vi "ContPreProc_old.vi"(8 "Step In":dbl, 10 "Compiler Settings":T1={"Python Path"=path "", "Main File"="makesequence.py", "Meta File"="makesequence.py", "Aux File"="C:\\Python27"}, 11 "Master Exp In":T2) -> (2 "Aux Pulse Out":T4, 3 "Main Pulse Out":T4)   [LabVIEW 2017]
uses:
  PulseControl.ctl
  Compiler/Params.ctl
  PulseCompiler/SequenceCluster.ctl
  controls/MasterExperiment.ctl
  PulseCompiler/CompilerSettings.ctl
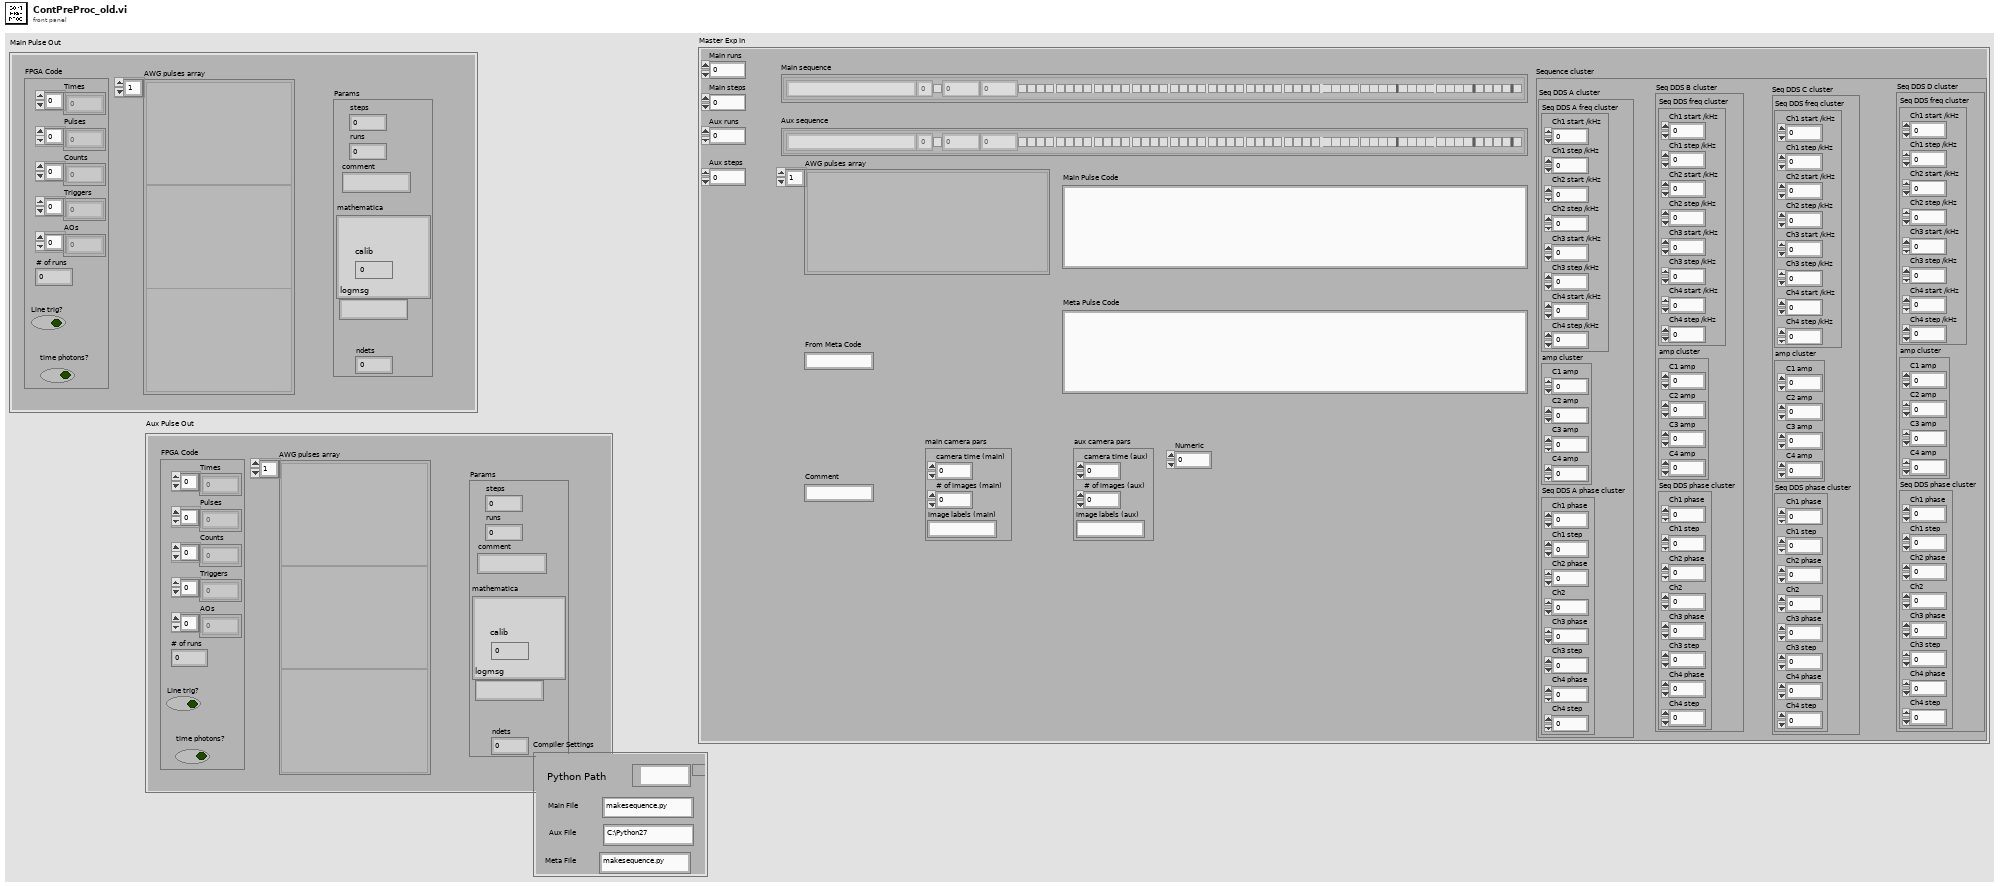
[diagram p1: front panel]
types:
  T1 = typedef "CompilerSettings.ctl" = cluster{"Python Path":path, "Main File":string, "Meta File":string, "Aux File":string}
  T2 = typedef "MasterExperiment.ctl" = cluster{"Main runs":dbl, "Numeric":dbl, "Main steps":dbl, "Aux runs":dbl, "Aux steps":dbl, "Main sequence":cluster{"Pulse name":string, "Pulse number":i32, "Enabled?":bool, "Time":dbl, "Step":dbl, "Pulse 0":bool, "Pulse 1":bool, "Pulse 2":bool, "Pulse 3":bool, "Pulse 4":bool, "Pulse 5":bool, "Pulse 6":bool, "Pulse 7":bool, "Pulse 8":bool, "Pulse 9":bool, "Pulse 10":bool, "Pulse 11":bool, "Pulse 12":bool, "Pulse 13":bool, "Pulse 14":bool, "Pulse 15":bool, "Pulse 16":bool, "Pulse 17":bool, "Pulse 18":bool, "Pulse 19":bool, "Pulse 20":bool, "Pulse 21":bool, "Pulse 22":bool, "Pulse 23":bool, "Pulse 24":bool, "Pulse 25":bool, "Pulse 26":bool, "Pulse 27":bool, "Pulse 28":bool, "Pulse 29":bool, "Pulse 30":bool, "Pulse 31":bool, "Pulse 32":bool, "Pulse 33":bool, "Pulse 34":bool, "Pulse 35":bool, "Pulse 36":bool, "Pulse 37":bool, "Pulse 38":bool, "Pulse 39":bool, "Count 0":bool, "Count 1":bool, "Count 2":bool, "Count 3":bool, "Count 4":bool, "Count 5":bool, "Count 6":bool, "Count 7":bool, "AO 0":bool, "AO 1":bool, "AO 2":bool, "AO 3":bool, "Trigger 0":bool}[], "Aux sequence":cluster{"Pulse name":string, "Pulse number":i32, "Enabled?":bool, "Time":dbl, "Step":dbl, "Pulse 0":bool, "Pulse 1":bool, "Pulse 2":bool, "Pulse 3":bool, "Pulse 4":bool, "Pulse 5":bool, "Pulse 6":bool, "Pulse 7":bool, "Pulse 8":bool, "Pulse 9":bool, "Pulse 10":bool, "Pulse 11":bool, "Pulse 12":bool, "Pulse 13":bool, "Pulse 14":bool, "Pulse 15":bool, "Pulse 16":bool, "Pulse 17":bool, "Pulse 18":bool, "Pulse 19":bool, "Pulse 20":bool, "Pulse 21":bool, "Pulse 22":bool, "Pulse 23":bool, "Pulse 24":bool, "Pulse 25":bool, "Pulse 26":bool, "Pulse 27":bool, "Pulse 28":bool, "Pulse 29":bool, "Pulse 30":bool, "Pulse 31":bool, "Pulse 32":bool, "Pulse 33":bool, "Pulse 34":bool, "Pulse 35":bool, "Pulse 36":bool, "Pulse 37":bool, "Pulse 38":bool, "Pulse 39":bool, "Count 0":bool, "Count 1":bool, "Count 2":bool, "Count 3":bool, "Count 4":bool, "Count 5":bool, "Count 6":bool, "Count 7":bool, "AO 0":bool, "AO 1":bool, "AO 2":bool, "AO 3":bool, "Trigger 0":bool}[], "AWG pulses array":variant[], "Main Pulse Code":string, "Meta Pulse Code":string, "Comment":string, "main camera pars":cluster{"camera time (main)":i32, "# of images (main)":i32, "image labels (main)":string}, "aux camera pars":cluster{"camera time (aux)":i32, "# of images (aux)":i32, "image labels (aux)":string}, "From Meta Code":string, "Sequence cluster":T3}
  T3 = typedef "SequenceCluster.ctl" = cluster{"Seq DDS A cluster":cluster{"Seq DDS A freq cluster":cluster{"Ch1 start /kHz":dbl, "Ch1 step /kHz":dbl, "Ch2 start /kHz":dbl, "Ch2 step /kHz":dbl, "Ch3 start /kHz":dbl, "Ch3 step /kHz":dbl, "Ch4 start /kHz":dbl, "Ch4 step /kHz":dbl}, "amp cluster":cluster{"C1 amp":dbl, "C2 amp":dbl, "C3 amp":dbl, "C4 amp":dbl}, "Seq DDS A phase cluster":cluster{"Ch1 phase":dbl, "Ch1 step":dbl, "Ch2 phase":dbl, "Ch2":dbl, "Ch3 phase":dbl, "Ch3 step":dbl, "Ch4 phase":dbl, "Ch4 step":dbl}}, "Seq DDS B cluster":cluster{"Seq DDS freq cluster":cluster{"Ch1 start /kHz":dbl, "Ch1 step /kHz":dbl, "Ch2 start /kHz":dbl, "Ch2 step /kHz":dbl, "Ch3 start /kHz":dbl, "Ch3 step /kHz":dbl, "Ch4 start /kHz":dbl, "Ch4 step /kHz":dbl}, "amp cluster":cluster{"C1 amp":dbl, "C2 amp":dbl, "C3 amp":dbl, "C4 amp":dbl}, "Seq DDS phase cluster":cluster{"Ch1 phase":dbl, "Ch1 step":dbl, "Ch2 phase":dbl, "Ch2":dbl, "Ch3 phase":dbl, "Ch3 step":dbl, "Ch4 phase":dbl, "Ch4 step":dbl}}, "Seq DDS C cluster":cluster{"Seq DDS freq cluster":cluster{"Ch1 start /kHz":dbl, "Ch1 step /kHz":dbl, "Ch2 start /kHz":dbl, "Ch2 step /kHz":dbl, "Ch3 start /kHz":dbl, "Ch3 step /kHz":dbl, "Ch4 start /kHz":dbl, "Ch4 step /kHz":dbl}, "amp cluster":cluster{"C1 amp":dbl, "C2 amp":dbl, "C3 amp":dbl, "C4 amp":dbl}, "Seq DDS phase cluster":cluster{"Ch1 phase":dbl, "Ch1 step":dbl, "Ch2 phase":dbl, "Ch2":dbl, "Ch3 phase":dbl, "Ch3 step":dbl, "Ch4 phase":dbl, "Ch4 step":dbl}}, "Seq DDS D cluster":cluster{"Seq DDS freq cluster":cluster{"Ch1 start /kHz":dbl, "Ch1 step /kHz":dbl, "Ch2 start /kHz":dbl, "Ch2 step /kHz":dbl, "Ch3 start /kHz":dbl, "Ch3 step /kHz":dbl, "Ch4 start /kHz":dbl, "Ch4 step /kHz":dbl}, "amp cluster":cluster{"C1 amp":dbl, "C2 amp":dbl, "C3 amp":dbl, "C4 amp":dbl}, "Seq DDS phase cluster":cluster{"Ch1 phase":dbl, "Ch1 step":dbl, "Ch2 phase":dbl, "Ch2":dbl, "Ch3 phase":dbl, "Ch3 step":dbl, "Ch4 phase":dbl, "Ch4 step":dbl}}}
  T4 = typedef "PulseControl.ctl" = cluster{"FPGA Code":cluster{"Times":u32[], "Pulses":u64[], "Counts":u8[], "Triggers":u8[], "AOs":u8[], "# of runs":i32, "Line trig?":bool, "time photons?":bool}, "AWG pulses array":variant[], "Params":T5}
  T5 = typedef "Params.ctl" = cluster{"steps":dbl, "runs":dbl, "comment":string, "mathematica":string, "calib":dbl, "logmsg":string, "ndets":dbl}
  T6 = cluster{"Pulse name":string, "Pulse number":i32, "Enabled?":bool, "Time":dbl, "Step":dbl, "Pulse 0":bool, "Pulse 1":bool, "Pulse 2":bool, "Pulse 3":bool, "Pulse 4":bool, "Pulse 5":bool, "Pulse 6":bool, "Pulse 7":bool, "Pulse 8":bool, "Pulse 9":bool, "Pulse 10":bool, "Pulse 11":bool, "Pulse 12":bool, "Pulse 13":bool, "Pulse 14":bool, "Pulse 15":bool, "Pulse 16":bool, "Pulse 17":bool, "Pulse 18":bool, "Pulse 19":bool, "Pulse 20":bool, "Pulse 21":bool, "Pulse 22":bool, "Pulse 23":bool, "Pulse 24":bool, "Pulse 25":bool, "Pulse 26":bool, "Pulse 27":bool, "Pulse 28":bool, "Pulse 29":bool, "Pulse 30":bool, "Pulse 31":bool, "Pulse 32":bool, "Pulse 33":bool, "Pulse 34":bool, "Pulse 35":bool, "Pulse 36":bool, "Pulse 37":bool, "Pulse 38":bool, "Pulse 39":bool, "Count 0":bool, "Count 1":bool, "Count 2":bool, "Count 3":bool, "Count 4":bool, "Count 5":bool, "Count 6":bool, "Count 7":bool, "AO 0":bool, "AO 1":bool, "AO 2":bool, "AO 3":bool, "Trigger 0":bool}[]
  T7 = cluster{"Pulse name":string, "Pulse number":i32, "Enabled?":bool, "Time":dbl, "Step":dbl, "digiouts":u64, "counts":u8, "AOs":u8, "triggers":u8}[]
  T8 = typedef "SinglePulse.ctl" = cluster{"enabled":bool, "string":string, "time":dbl, "step":dbl, "dio":dbl, "count":dbl, "trigger":dbl, "AO":dbl}
  T9 = cluster{"Times":u32[], "Pulses":u64[], "Counts":u8[], "Triggers":u8[], "AOs":u8[], "Aux runs":dbl, bool, bool}
  T10 = cluster{"Times":u32[], "Pulses":u64[], "Counts":u8[], "Triggers":u8[], "AOs":u8[], "Main runs":dbl, bool, bool}
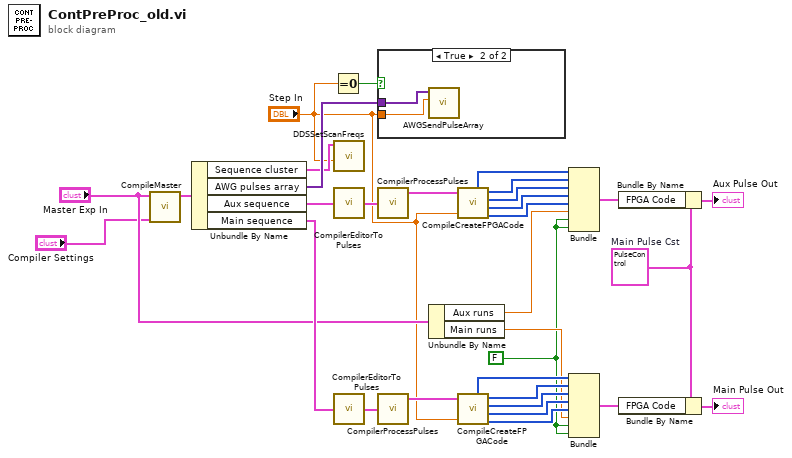
[diagram p0: block diagram]
diagram:
  w8 = FALSE
  w7 = T4 {"FPGA Code"={"Times"=[], "Pulses"=[], "Counts"=[], "Triggers"=[], "AOs"=[], "# of runs"=0, "Line trig?"=FALSE, "time photons?"=FALSE}, "AWG pulses array"=[], "Params"={"steps"=0.0, "runs"=0.0, "comment"="", "mathematica"="", "calib"=0.0, "logmsg"="", "ndets"=0.0}}  # Main Pulse Cst
  n1 = call "CompileMaster.vi"("Compiler Settings"="Compiler Settings", "Master Exp In"="Master Exp In") -> ("Master Exp Out"=w22:T2)  [unwired: 3 in, 2 out]
  n2 = Unbundle By Name(w22) -> ("Sequence cluster"=w2:T3, "AWG pulses array"=w4:variant[], "Aux sequence"=w18:T6, "Main sequence"=w21:T6)
  n3 = Equal To 0?(x="Step In") -> (x = 0?=w3:bool)
  n4 = call "DDSSetScanFreqs.vi"("Step number"="Step In", "Sequence cluster 2"=w2) -> ()  [unwired: 5 in, 2 out]
  n5 = call "CompilerEditorToPulses.vi"("Seq In"=w18) -> ("Combined pulse array"=w17:T7)
  n6 = call "CompilerEditorToPulses.vi"("Seq In"=w21) -> ("Combined pulse array"=w23:T7)
  n7 = case shown="True" w3 {
    tunnel: "Step In" -> [_ w33]
    tunnel: w4 -> [_ w32]
    frame False {
    }
    frame True {
      n8 = call "AWGSendPulseArray.vi"("Step Number"=w33, "AWG pulses array"=w32) -> ()  [unwired: 9 in, 1 out]
    }
  }
  n9 = call "CompilerProcessPulses.vi"("Pulse Seq In"=w17) -> ("Pulse Seq Out"=w15:T8[])  [unwired: 2 out]
  n10 = call "CompilerProcessPulses.vi"("Pulse Seq In"=w23) -> ("Pulse Seq Out"=w24:T8[])  [unwired: 2 out]
  n11 = Unbundle By Name("Master Exp In") -> ("Aux runs"=w9:dbl, "Main runs"=w16:dbl)
  n12 = call "CompileCreateFPGACode.vi"("Enabled pulse array 2"=w15, "step #"="Step In") -> ("Pulses"=w13:u64[], "Times"=w14:u32[], "Counts"=w12:u8[], "Triggers"=w11:u8[], "AOs"=w10:u8[])  [unwired: 1 in, 1 out]
  n13 = call "CompileCreateFPGACode.vi"("Enabled pulse array 2"=w24, "step #"="Step In") -> ("Pulses"=w27:u64[], "Times"=w29:u32[], "Counts"=w28:u8[], "Triggers"=w30:u8[], "AOs"=w31:u8[])  [unwired: 1 in, 1 out]
  n14 = Bundle("Times"=w14, "Pulses"=w13, "Counts"=w12, "Triggers"=w11, "AOs"=w10, "Aux runs"=w9, w8, w8) -> (w5:T9)  [unwired: 1 in]
  n15 = Bundle("Times"=w29, "Pulses"=w27, "Counts"=w28, "Triggers"=w30, "AOs"=w31, "Main runs"=w16, w8, w8) -> (w26:T10)  [unwired: 1 in]
  n16 = Bundle By Name(cluster=w7, "FPGA Code"=w5) -> (→"Aux Pulse Out":T4)
  n17 = Bundle By Name(cluster=w7, "FPGA Code"=w26) -> (→"Main Pulse Out":T4)
